vi "T_step_mischer.vi"   [LabVIEW 2019]
uses:
  Global/Global Variables/global.vi
  Instrument_Setup.vi
  Global/Global Variables/Data_Display_global.vi
types:
  T1 = typedef "LS372-Cluster.ctl" = cluster{"Activate Tsweep":bool, "Setpoint - Manual":dbl, "Rate (K/min)":dbl, "Update Lakeshores":bool, "Still Heater":bool, "Still Power (mW)":dbl, "Manual Heater":bool, "Manual Heater  (mW) ":dbl, "Heater Range":dbl, "P (Gain)":dbl, "I (Reset)":dbl, "D (Rate)":dbl, "Heater Power (mW)":dbl, "MC Thermometer":u16, "MC Temperature":dbl, "LS372-T1":dbl, "LS372 -T2":dbl, "LS372-R1 ":dbl, "LS372-R2":dbl, "LS372-T3":dbl, "LS372-T4":dbl, "LS372-R3 ":dbl, "LS372-R4 \n\n\n\n":dbl, "LS372-T5":dbl, "LS372-T6":dbl, "LS372-R5":dbl, "LS372-R6 ":dbl, "Still Power ist":dbl, "Set Temperatur Sweep main":bool, "Setpoint ist":dbl, "Disable Heater":bool}
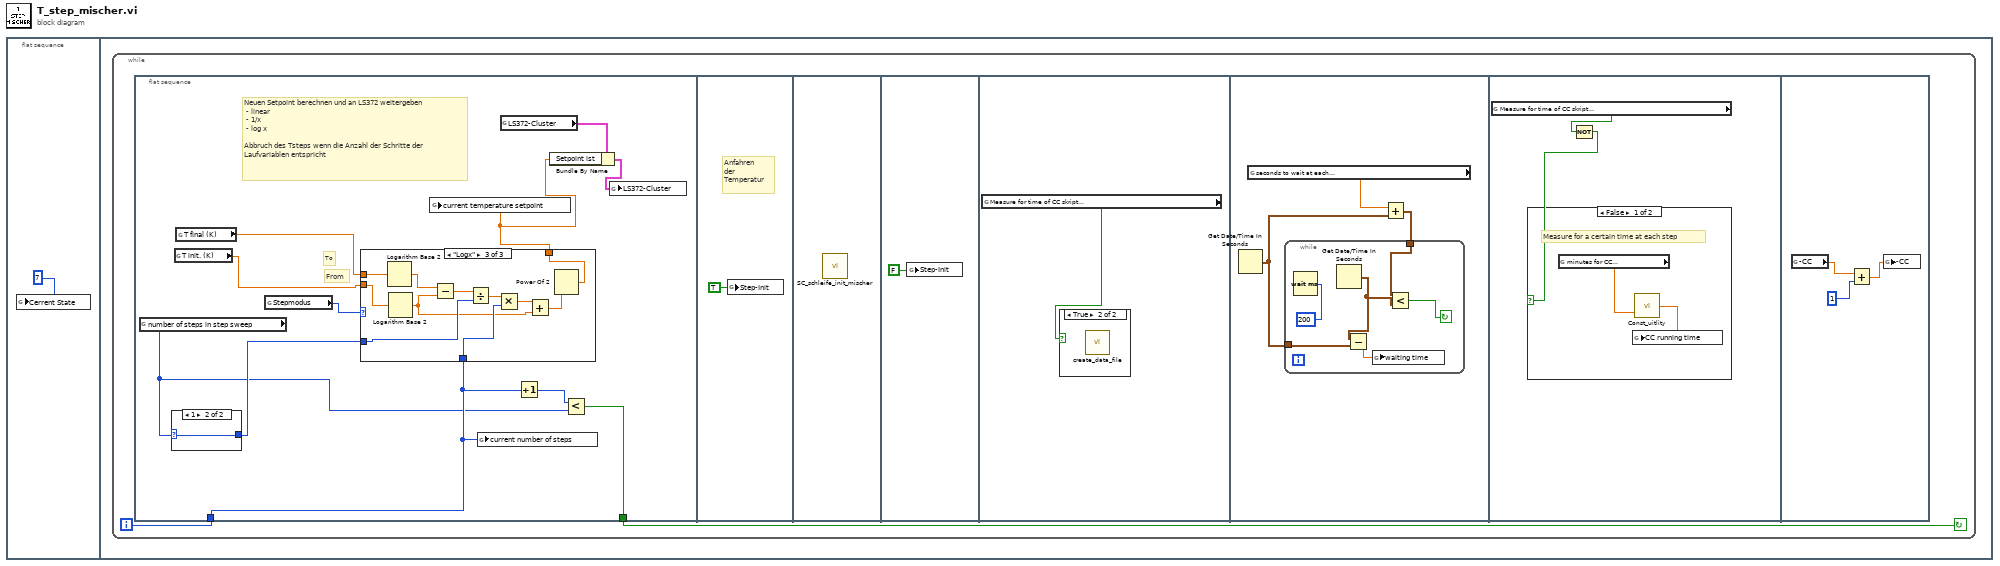
[diagram p0: block diagram]
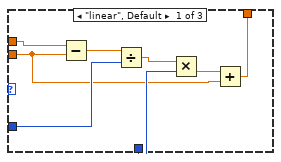
[diagram p2: hidden frame]
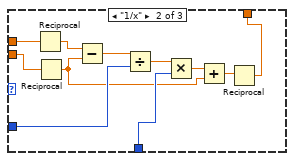
[diagram p3: hidden frame]
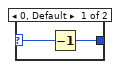
[diagram p4: hidden frame]
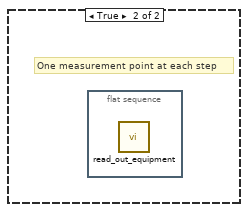
[diagram p6: hidden frame]
diagram:
  n1 = flat-sequence {
    frame #0 {
      n2 = global write "global.vi" "Cerrent State"(7) -> ()
    }
    frame #1 {
      n3 = while {
        i -> [w3]
        stop <- w2 continue-if-true
        n4 = flat-sequence {
          tunnel: w3 -> [w10]
          tunnel: [w7] -> w2
          frame #0 {
            # "From"
            # "To"
            # "Neuen Setpoint berechnen und an LS372 weitergeben\n - linear\n - 1/x\n - log x\n\nAbbruch des Tsteps wenn die Anzahl der Schritte der \nLaufvariablen entspricht"
            n5 = global read "global.vi" "number of steps in step sweep"() -> (w8:i32)
            n6 = case shown="1" w8 {
              selector: w8 -> [w46 w47]
              tunnel: [w45 w47] -> w11
              frame 0, Default {
                n7 = Decrement(x=w46) -> (x-1=w45:i32)
              }
              frame 1 {
              }
            }
            n8 = global read "global.vi" "T init. (K)"() -> (w12:dbl)
            n9 = global read "global.vi" "T final (K)"() -> (w13:dbl)
            n10 = global read "Instrument_Setup.vi" "Stepmodus"() -> (w14:enum16{"linear", "1/x", "Logx"})
            n11 = case shown="\"Logx\"" w14 {
              tunnel: w13 -> [w22 w33 w44]
              tunnel: w12 -> [w16 w32 w43]
              tunnel: w11 -> [w20 w29 w40]
              tunnel: w10 -> [w18 w27 w38]
              tunnel: [w15 w23 w34] -> w4
              frame "linear", Default {
                n12 = Subtract(x=w22, y=w16) -> (x-y=w21:dbl)
                n13 = Divide(x=w21, y=w20) -> (x/y=w19:dbl)
                n14 = Multiply(x=w19, y=w18) -> (x*y=w17:dbl)
                n15 = Add(x=w17, y=w16) -> (x+y=w15:dbl)
              }
              frame "1/x" {
                n16 = Reciprocal(x=w33) -> (1/x=w31:dbl)
                n17 = Reciprocal(x=w32) -> (1/x=w25:dbl)
                n18 = Subtract(x=w31, y=w25) -> (x-y=w30:dbl)
                n19 = Divide(x=w30, y=w29) -> (x/y=w28:dbl)
                n20 = Multiply(x=w28, y=w27) -> (x*y=w26:dbl)
                n21 = Add(x=w26, y=w25) -> (x+y=w24:dbl)
                n22 = Reciprocal(x=w24) -> (1/x=w23:dbl)
              }
              frame "Logx" {
                n23 = Logarithm Base 2(1:w44) -> (0:w42:dbl)
                n24 = Logarithm Base 2(1:w43) -> (0:w36:dbl)
                n25 = Subtract(x=w42, y=w36) -> (x-y=w41:dbl)
                n26 = Divide(x=w41, y=w40) -> (x/y=w39:dbl)
                n27 = Multiply(x=w39, y=w38) -> (x*y=w37:dbl)
                n28 = Add(x=w37, y=w36) -> (x+y=w35:dbl)
                n29 = Power Of 2(x=w35) -> (2^x=w34:dbl)
              }
            }
            n30 = global write "Data_Display_global.vi" "current temperature setpoint"(w4) -> ()
            n31 = global write "Data_Display_global.vi" "current number of steps"(w10) -> ()
            n32 = global read "Data_Display_global.vi" "LS372-Cluster"() -> (w6:T1)
            n33 = Increment(x=w10) -> (x+1=w9:i32)
            n34 = Bundle By Name(cluster=w6, "Setpoint ist"=w4) -> (w5:T1)
            n35 = Less?(x=w9, y=w8) -> (x < y?=w7:bool)
            n36 = global write "Data_Display_global.vi" "LS372-Cluster"(w5) -> ()
          }
          frame #1 {
            # "Anfahren \nder \nTemperatur"
            n37 = global write "global.vi" "Step-Init"(TRUE) -> ()
          }
          frame #2 {
            n38 = call "SC_schleife_init_mischer.vi"() -> ()  [unwired: 4 in]
          }
          frame #3 {
            n39 = global write "global.vi" "Step-Init"(FALSE) -> ()
          }
          frame #4 {
            n40 = global read "Instrument_Setup.vi" "Measure for time of CC skript\nat each field step point"() -> (w50:bool)
            n41 = case shown="True" w50 {
              frame False {
              }
              frame True {
                n42 = call "create_data_file.vi"() -> ()  [unwired: 3 in]
              }
            }
          }
          frame #5 {
            n43 = Get Date/Time In Seconds() -> (seconds since 1Jan1904=w51:timestamp)
            n44 = global read "Instrument_Setup.vi" "seconds to wait at each\nfield step in a step sweep"() -> (w53:dbl)
            n45 = Add(x=w53, y=w51) -> (x+y=w52:timestamp)
            n46 = while {
              tunnel: w52 -> [w55]
              tunnel: w51 -> [w58]
              stop <- w54 continue-if-true
              n47 = Wait (ms)(milliseconds to wait=200) -> ()  [unwired: 1 out]
              n48 = Get Date/Time In Seconds() -> (seconds since 1Jan1904=w56:timestamp)
              n49 = Subtract(x=w56, y=w58) -> (x-y=w57:dbl)
              n50 = global write "Data_Display_global.vi" "waiting time"(w57) -> ()
              n51 = Less?(x=w56, y=w55) -> (x < y?=w54:bool)
            }
          }
          frame #6 {
            n52 = global read "Instrument_Setup.vi" "Measure for time of CC skript\nat each field step point"() -> (w61:bool)
            n53 = Not(x=w61) -> (.not. x?=w60:bool)
            n54 = case shown="False" w60 {
              frame False {
                # "Measure for a certain time at each step"
                n55 = global read "Instrument_Setup.vi" "minutes for CC\nto run"() -> (w63:dbl)
                n56 = call "Const_uitlity.vi"("Duration"=w63) -> ("Minutes passed"=w62:dbl)  [unwired: 1 in]
                n57 = global write "Data_Display_global.vi" "CC running time"(w62) -> ()
              }
              frame True {
                # "One measurement point at each step"
                n58 = flat-sequence {
                  frame #0 {
                    n59 = call "read_out_equipment.vi"() -> ()  [unwired: 1 in]
                  }
                }
              }
            }
          }
          frame #7 {
            n60 = global read "global.vi" "-CC"() -> (w66:dbl)
            n61 = Add(x=w66, y=1) -> (x+y=w64:dbl)
            n62 = global write "global.vi" "-CC"(w64) -> ()
          }
        }
      }
    }
  }
